vi "test udp++.vi"() -> ()   [LabVIEW 2017]
uses:
  <vilib>/Platform/TimedLoop/XDataNode/timing_clust.ctl
  <vilib>/Platform/TimedLoop/XDataNode/nitl_modes.ctl
  <vilib>/Platform/TimedLoop/XDataNode/wakeup.ctl
  16e1070c-7dc9-4f03-9a7c-c4bc31601776.vi
  dd86c118-00dc-4621-9a13-23dbe0247810.vi
  <vilib>/Utility/High Resolution Relative Seconds.vi
  16e1070c-7dc9-4f03-9a7c-c4bc31601776.vi/c01658a1-883f-489e-b376-c551e55a1c83.vi
  dd86c118-00dc-4621-9a13-23dbe0247810.vi/f576cfcf-0274-437d-9d31-e81457e56e77.vi
  <userlib>/_NEVSTOP/GlobalStop/_gStop.vi
  SplitUDPPacks.vi
  <userlib>/_OpenG.lib/comparison/comparison.llb/Data Changed__ogtk.vi
  <userlib>/_OpenG.lib/comparison/comparison.llb/I32 Changed__ogtk.vi
  <vilib>/Platform/TimedLoop/XDataNode/XDataNode.xnode
  <vilib>/Platform/TimedLoop/XDataNode/XDNodeRunTimeDep.lvlib
  <userlib>/_NEVSTOP/GlobalStop/GSTOP.lvlib
panel:
  out "sumcheck 2":dbl[](array[numeric])
  out "sumcheck":dbl
  out "# Count":i64[](array[numeric])
  out "time diff(s)":dbl
  in  "Numeric":i32=500
  out "Array":sgl[](array[numeric])
  out "接收控制指令":sgl[](array[numeric])
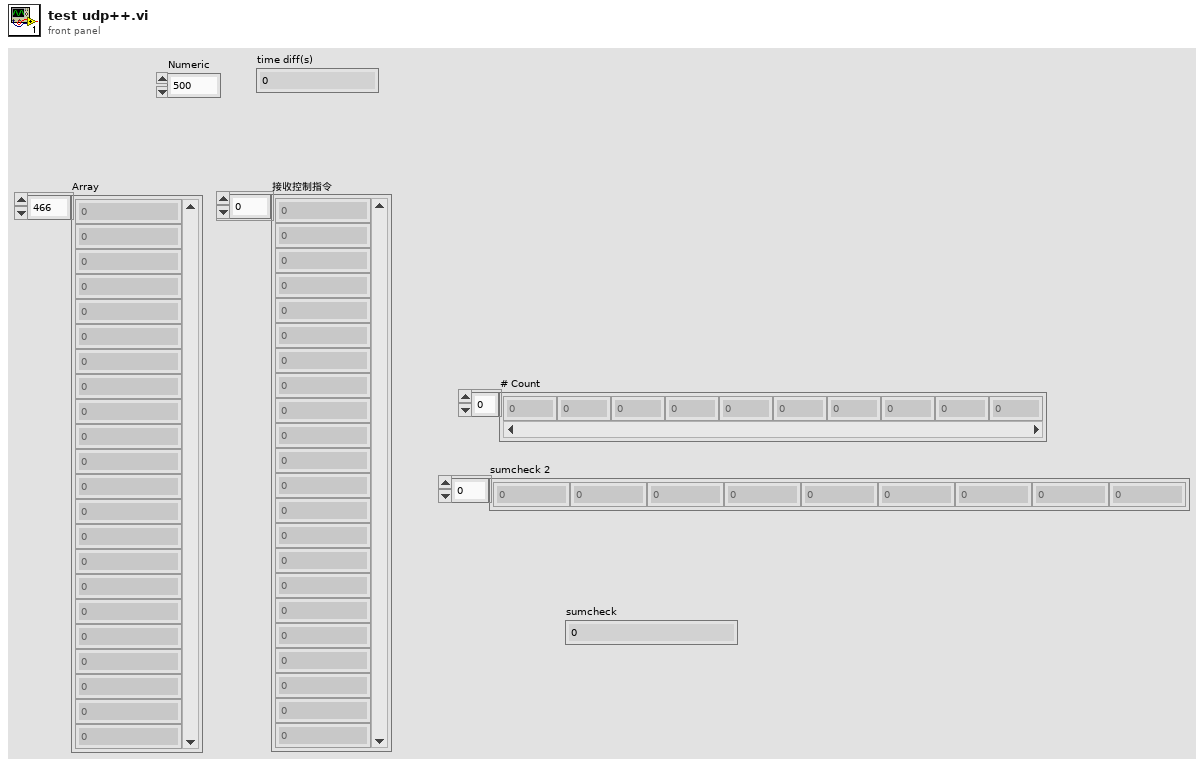
[diagram p1: front panel]
types:
  T1 = cluster{"本地IP":string, "本地端口":u16, "远程IP":string, "远程端口":u16}
  T2 = typedef "XDNodeRunTimeDep.lvlib/timing_clust.ctl" = cluster{"Expected End [f-1]":u64, "Actual End [f-1]":u64, "Finished Late? [f-1]":bool, "Expected End [i-1]":u64, "Actual End [i-1]":u64, "Finished Late? [i-1]":bool, "Expected Start [i]":u64, "Actual Start [i]":u64, "Expected Start [f]":u64, "Actual Start [f]":u64, "Source Name":string, "Structure Name":string, "Period":i64, "Deadline":i64, "Offset":i64, "Start":i64, "Priority":i32, "Timeout":i32, "Mode":T3, "Wakeup Reason":T4, "Error":errorcluster, "Source Type":string, "Secondary Source Type":string, "Global End Time":u64, "Global Start Time":u64, "Frame Duration":u64, "Iteration Duration":u64, "Assigned CPU":i32, "I/O Scan Engine Mode":u32}
  T3 = typedef "XDNodeRunTimeDep.lvlib/nitl_modes.ctl" = enum32{"No Change", "Process missed periods, maintain original phase", "Discard missed periods, maintain original phase", "Process missed periods, ignore original phase", "Discard missed periods, ignore original phase"}
  T4 = typedef "XDNodeRunTimeDep.lvlib/wakeup.ctl" = enum32{"Normal", "Aborted", "Asynchronous wakeup", "Timing source error", "Timed loop error", "Timeout"}
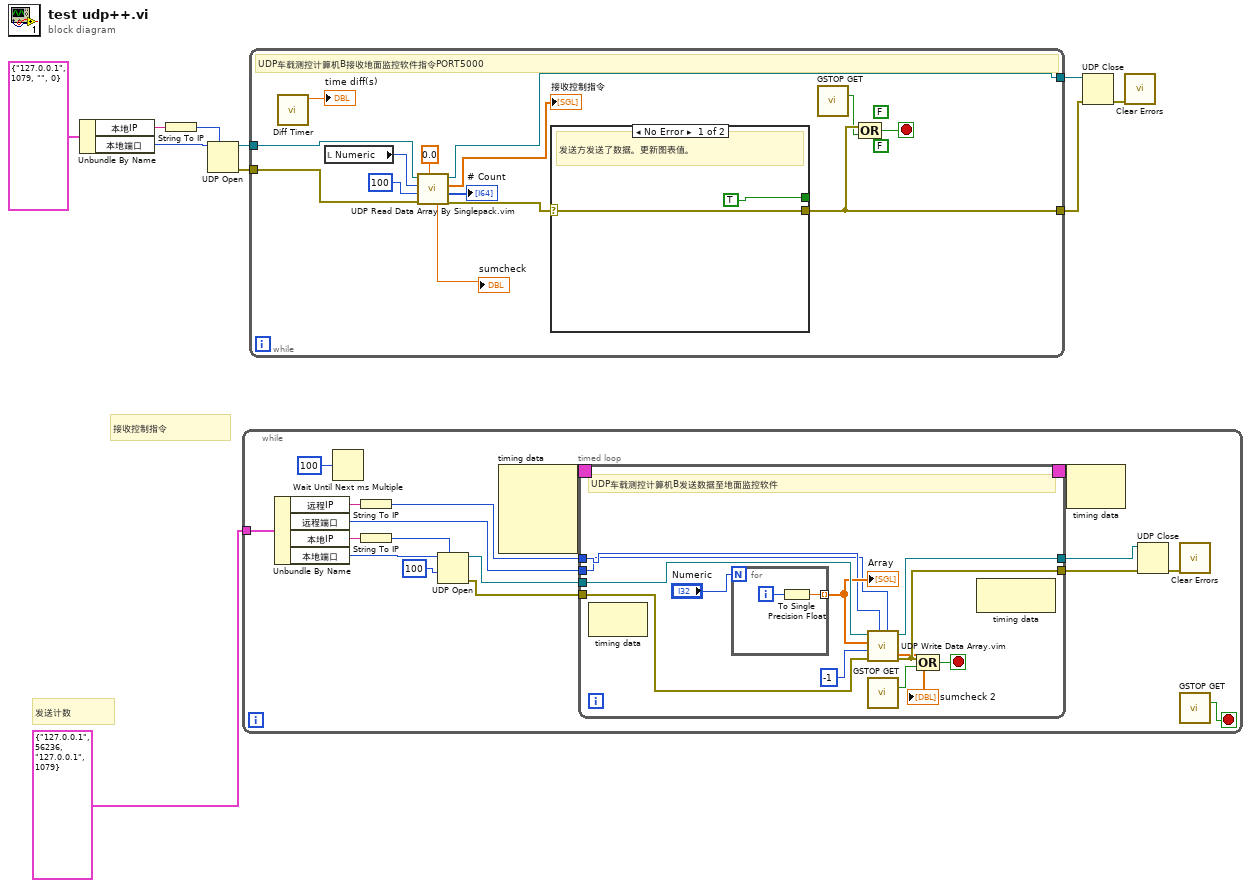
[diagram p0: block diagram]
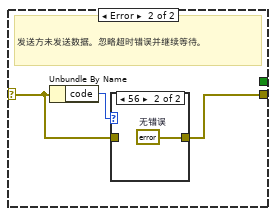
[diagram p2: hidden frame]
diagram:
  # "发送计数"
  # "接收控制指令"
  n1 = Unbundle By Name(T1 {"本地IP"="127.0.0.1", "本地端口"=1079, "远程IP"="", "远程端口"=0} ("UDP配置")) -> ("本地IP"=w3:string, "本地端口"=w2:u16)
  n2 = String To IP(1:w3) -> (0:w10:u32)
  n3 = UDP Open(7:w10, 11:w2) -> (port=w9:refnum<k16>, 0:w8:errorcluster)  [unwired: 3 in, 1 out]
  n4 = while {
    tunnel: T1 {"本地IP"="127.0.0.1", "本地端口"=56236, "远程IP"="127.0.0.1", "远程端口"=1079} ("UDP配置") -> [w15]
    stop <- w19 stop-if-true
    n5 = Unbundle By Name(w15) -> ("远程IP"=w12:string, "远程端口"=w11:u16, "本地IP"=w13:string, "本地端口"=w14:u16)
    n6 = Wait Until Next ms Multiple(millisecond multiple=u32 100 ("毫秒倍数")) -> ()  [unwired: 1 out]
    n7 = String To IP(1:w12) -> (0:w21:u32)
    n8 = String To IP(1:w13) -> (0:w23:u32)
    n9 = UDP Open(7:w23, 9:100 ("超时毫秒(25000)"), 11:w14) -> (port=w25:refnum<k16>, 0:w24:errorcluster)  [unwired: 2 in, 1 out]
    n10 = node-c288() -> (w27:T2)  [unwired: 4 in]
    n11 = timed-loop {
      tunnel: [w36] -> w18
      tunnel: w25 -> [w39]
      tunnel: w24 -> [w37]
      tunnel: [w38] -> w17
      tunnel: w11 -> [w30]
      timing: w27 -> [_]
      timing-out: [_] -> w26
      tunnel: w21 -> [w31]
      stop <- w35 stop-if-true
      # "UDP车载测控计算机B发送数据至地面监控软件"
      n12 = node-c288() -> ()  [unwired: 1 in, 1 out]
      n13 = for {
        N: "Numeric" -> [_]
        tunnel: [w40] -> w32 mode=indexing
        i -> [w41]
        n14 = To Single Precision Float(number=w41) -> (single precision float=w40:sgl)
      }
      "Array" <- w32
      n15 = call "UDP Write Data Array.vim"("port or service name"=w30, "address"=w31, "error in (no error)"=w37, "超时毫秒(25000)"=-1, "Data"=w32, "UDP Network Connection in"=w39) -> ("error out"=w36:errorcluster, "UDP Network Connection out"=w38:refnum<k16>, "checksum"=→"sumcheck 2":dbl[])  [unwired: 3 in]
      n16 = call <userlib>:"GSTOP GET.vi"() -> ("stop"=w34:bool)  [unwired: 14 in, 1 out]
      n17 = Compound Arithmetic op=OR ("复合运算")(w36, w34) -> (w35:bool)
      n18 = node-c288() -> ()  [unwired: 1 in, 1 out]
    }
    n19 = node-c288(w26) -> ()  [unwired: 1 out]
    n20 = UDP Close(connection ID=w17, 8:w18) -> (error out=w16:errorcluster)  [unwired: 1 out]
    n21 = call <vilib>:"Clear Errors.vi"("error in (no error)"=w16) -> ()  [unwired: 5 in, 2 out]
    n22 = call <userlib>:"GSTOP GET.vi"() -> ("stop"=w19:bool)  [unwired: 14 in, 1 out]
  }
  n23 = while {
    tunnel: w9 -> [w59]
    tunnel: [w57] -> w6
    tunnel: w8 -> [w58]
    tunnel: [w56] -> w7
    stop <- w55 stop-if-true
    (unwired) FALSE ("reset value")
    (unwired) FALSE ("reset")
    # "UDP车载测控计算机B接收地面监控软件指令PORT5000"
    n24 = call "Diff Timer.vi"() -> ("time diff(s)"=→"time diff(s)":dbl)  [unwired: 10 in, 1 out]
    n25 = local read "Numeric"() -> (w50:i32)
    n26 = call "UDP Read Data Array By Singlepack.vim"("Data Type(dbl)"=sgl 0.0, "error in (no error)"=w58, "超时毫秒(25000)"=100 ("timeout ms (25000)"), "total size"=w50, "UDP Network Connection in"=w59) -> ("error out"=w53:errorcluster, "# Count"=→"# Count":i64[], "Array"=→"接收控制指令":sgl[], "UDP Network Connection out"=w57:refnum<k16>, "checksum"=→"sumcheck":dbl)  [unwired: 2 in]
    n27 = case shown="No Error" w53 {
      selector: w53 -> [w61 w63]
      tunnel: [w61 w62] -> w56
      tunnel: [TRUE ("wifi_KongZ") _] -> _
      frame No Error {
        # "发送方发送了数据。更新图表值。"
      }
      frame Error {
        # "发送方未发送数据。忽略超时错误并继续等待。"
        n28 = Unbundle By Name(w63) -> ("code"=w64:i32)
        n29 = case shown="56" w64 {
          tunnel: w63 -> [w65 _]
          tunnel: [w65 w66] -> w62
          frame Default {
          }
          frame 56 {
            w66 = errorcluster {"status"=FALSE, "code"=0, "source"=""}  # 无错误
          }
        }
      }
    }
    n30 = call <userlib>:"GSTOP GET.vi"() -> ("stop"=w51:bool)  [unwired: 14 in, 1 out]
    n31 = Compound Arithmetic op=OR ("复合运算")(w56, w51) -> (w55:bool)
  }
  n32 = UDP Close(connection ID=w6, 8:w7) -> (error out=w5:errorcluster)  [unwired: 1 out]
  n33 = call <vilib>:"Clear Errors.vi"("error in (no error)"=w5) -> ()  [unwired: 5 in, 2 out]
